vi "Lines LoadMatrixOfSessions.vi"(7 "Annotation Seperator(#)":string="#", 8 "error in (no error)":errorcluster, 9 "Session Name(Rxp)":string, 10 "Array in":string[](array[string]), 11 "Lines":string[](array[string])) -> (0 "error out":errorcluster, 2 "Array out":string[][](array[string]), 3 "Config Text List out":string[](array[string]))   [LabVIEW 2017, in "ini_configuration.lvlib"]
uses:
  ini_configuration.lvlib
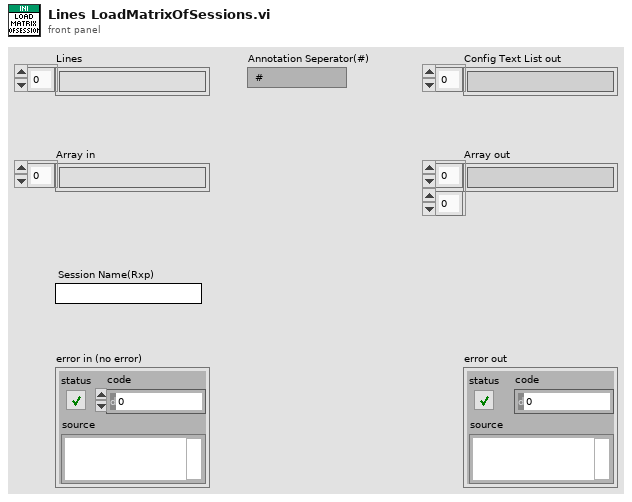
[diagram p1: front panel]
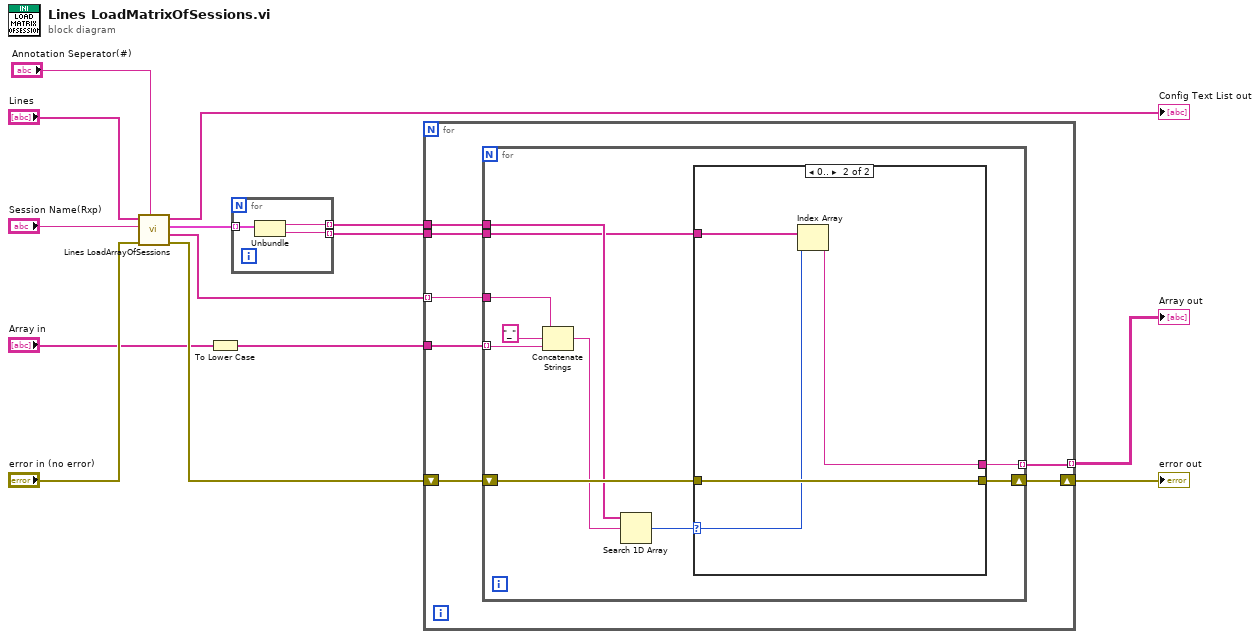
[diagram p0: block diagram]
diagram:
  n1 = call "Lines LoadArrayOfSessions.vi"("Annotation Seperator(#)"="Annotation Seperator(#)", "error in (no error)"="error in (no error)", "Session Name"="Session Name(Rxp)", "Lines"="Lines") -> ("error out"=w12:errorcluster, "Matched Sessions"=w7:string[], "String Config Group"=w8:cluster{"Key":string, "Value":string}[], "Config Text List out"=→"Config Text List out":string[])  [unwired: 4 in]
  n2 = To Lower Case(string="Array in") -> (all lower case string=w2:string[])
  n3 = for {
    tunnel: w8 -> [w17] mode=indexing
    tunnel: [w16] -> w9 mode=indexing
    tunnel: [w15] -> w10 mode=indexing
    n4 = Unbundle(w17) -> ("Key"=w16:string, "Value"=w15:string)
  }
  n5 = for {
    tunnel: w9 -> [w22]
    tunnel: w7 -> [w21] mode=indexing
    tunnel: w2 -> [w20]
    shift-right: [w24] -> w5
    shift-left: w12 -> [w23]
    tunnel: [w19] -> w4 mode=indexing
    tunnel: w10 -> [w18]
    n6 = for {
      shift-right: [w34] -> w24
      shift-left: w23 -> [w33]
      tunnel: w22 -> [w30]
      tunnel: w21 -> [w27]
      tunnel: [w32] -> w19 mode=indexing
      tunnel: w20 -> [w28] mode=indexing
      tunnel: w18 -> [w25]
      n7 = Concatenate Strings(w27, "_" ("string"), w28) -> (w29:string)
      n8 = Search 1D Array(1D array=w30, element=w29) -> (index of element=w26:i32)  [unwired: 1 in]
      n9 = case shown="0.." w26 {
        selector: w26 -> [_ w37]
        tunnel: [w35 w39] -> w34
        tunnel: w33 -> [w35 w39]
        tunnel: [_ w36] -> w32
        tunnel: w25 -> [_ w38]
        frame Default {
        }
        frame 0.. {
          n10 = Index Array(array=w38, index=w37) -> (element=w36:string)
        }
      }
    }
  }
  "error out" <- w5
  "Array out" <- w4
